vi "PIZWithdraw.vi"() -> ()   [LabVIEW 2014]
uses:
  <vilib>/rvi/Emulation/niFpgaSctlEmulationGetInTimedLoop.vi
  <vilib>/rvi/Emulation/niFpgaProcessEmulError.vi
  <vilib>/rvi/Emulation/niFpgaGetClockAttributes.vi
  <vilib>/rvi/Emulation/niFpgaEmulationReportErrorSimple.vi
  <vilib>/rvi/eio/common/nirviEmuTemplateMethod_errors.vi
  <vilib>/rvi/Emulation/niFpgaCriticalErrorInLSC.vi
  <vilib>/eio/EIONode/EIONode.xnode
panel:
  out "PIZPos?":i16
  out "preCurrIndex":i16
  out "Withdrawn?":bool
  in  "Sleep ms":i16
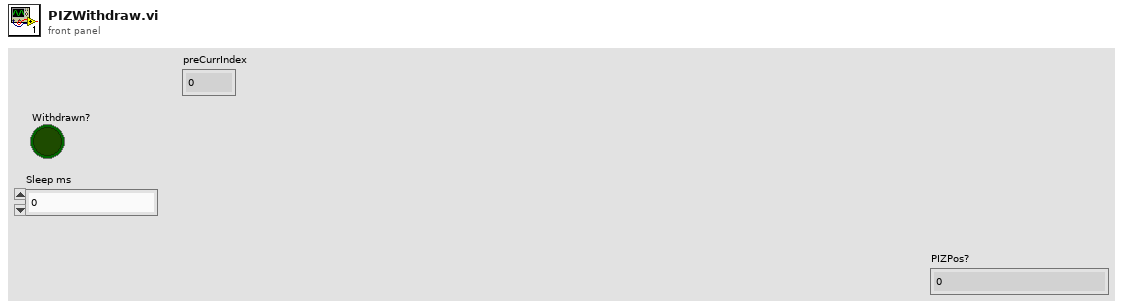
[diagram p1: front panel]
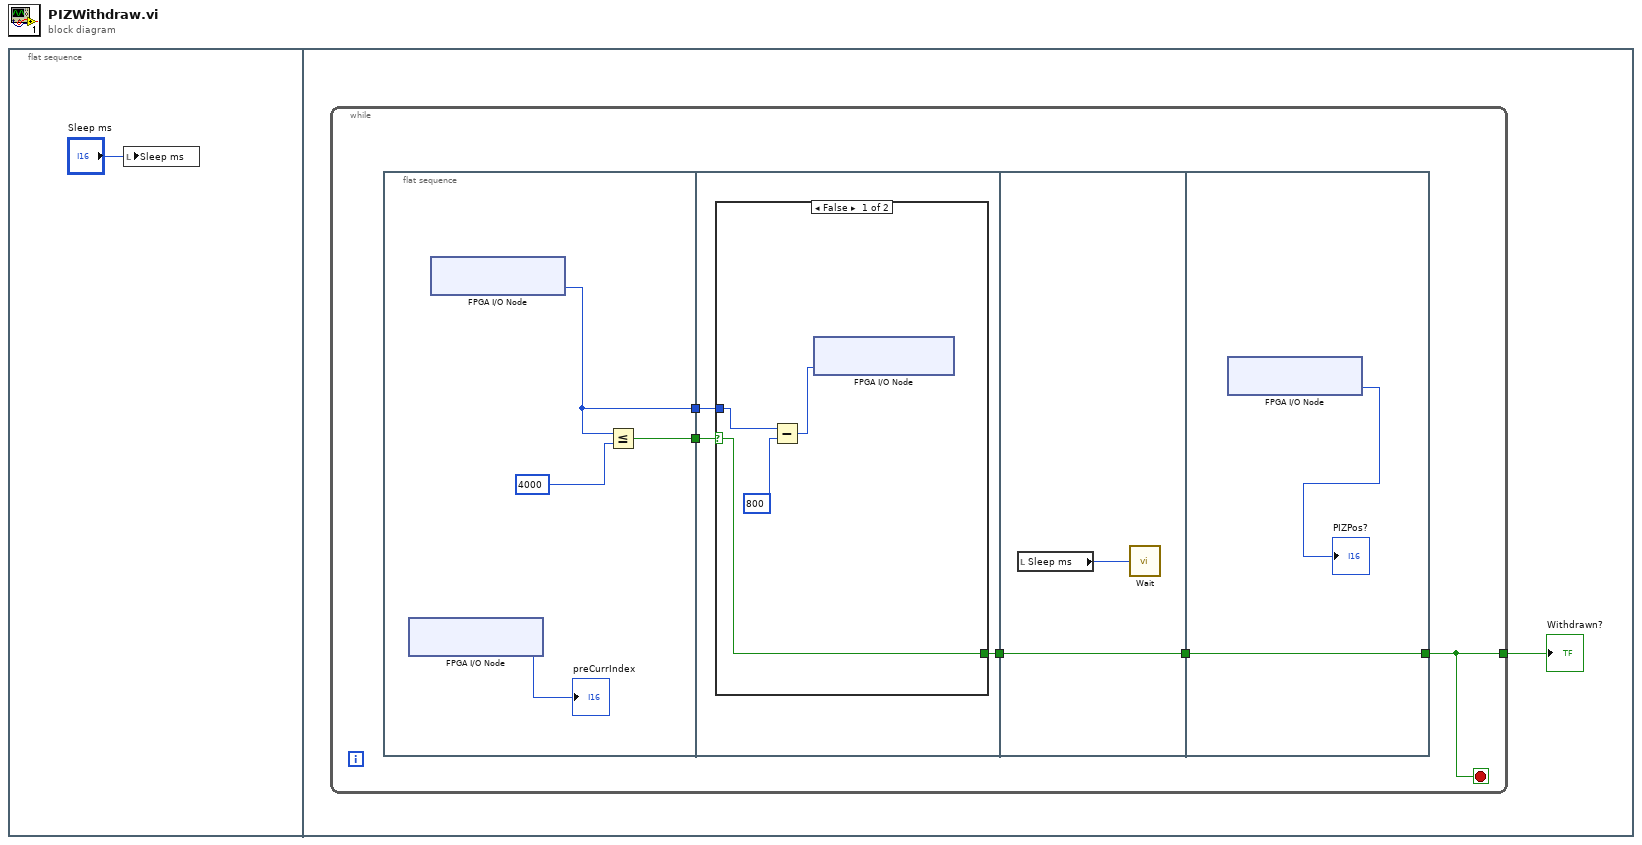
[diagram p0: block diagram]
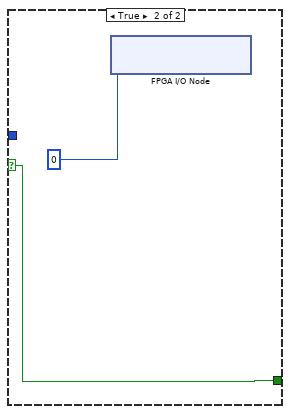
[diagram p2: hidden frame]
diagram:
  n1 = flat-sequence {
    frame #0 {
      n2 = local write "Sleep ms"("Sleep ms") -> ()
    }
    frame #1 {
      n3 = while {
        tunnel: [w4] -> w2
        stop <- w4 stop-if-true
        n4 = flat-sequence {
          tunnel: [w10] -> w7
          tunnel: [w9] -> w6
          tunnel: w7 -> [w14]
          tunnel: w6 -> [w13]
          tunnel: [w12] -> w5
          tunnel: w5 -> [w21]
          tunnel: [w21] -> w3
          tunnel: [w24] -> w4
          tunnel: w3 -> [w24]
          frame #0 {
            n5 = xnode "FPGA I/O Node"() -> ("Connector0/AI1"=→"preCurrIndex":i16)  [unwired: 1 in, 1 out]
            n6 = xnode "FPGA I/O Node"() -> ("Connector0/AI0"=w9:i16)  [unwired: 1 in, 1 out]
            n7 = Less Or Equal?(x=w9, y=i16 4000) -> (x <= y?=w10:bool)
          }
          frame #1 {
            n8 = case shown="False" w14 {
              selector: w14 -> [w15 w19]
              tunnel: w13 -> [w18 _]
              tunnel: [w15 w19] -> w12
              frame False {
                n9 = Subtract(x=w18, y=i16 800) -> (x-y=w16:i16)
                n10 = xnode "FPGA I/O Node"("Connector0/AO0"=w16) -> ()  [unwired: 1 in, 1 out]
              }
              frame True {
                n11 = xnode "FPGA I/O Node"("Connector0/AO0"=i16 0) -> ()  [unwired: 1 in, 1 out]
              }
            }
          }
          frame #2 {
            n12 = local read "Sleep ms"() -> (w22:i16)
            n13 = call "Wait"("Count(mSec)"=w22) -> ()  [unwired: 1 out]
          }
          frame #3 {
            n14 = xnode "FPGA I/O Node"() -> ("Connector0/AI0"=→"PIZPos?":i16)  [unwired: 1 in, 1 out]
          }
        }
      }
      "Withdrawn?" <- w2
    }
  }
